vi "三个数中的最大最小数.vi"(1 "c":dbl, 2 "b":dbl, 3 "a":dbl) -> (0 "max":dbl)   [LabVIEW 2012]
doc: "功能：\n\n求给定三个数中的最大、最小值。\n\ncsxcs_366创建"
panel:
  out "min":dbl
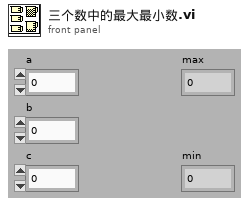
[diagram p1: front panel]
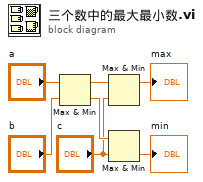
[diagram p0: block diagram]
diagram:
  n1 = Max & Min(x="a", y="b") -> (max(x,y)=w5:dbl, min(x,y)=w4:dbl)
  n2 = Max & Min(x=w5, y="c") -> (max(x,y)=→"max":dbl)  [unwired: 1 out]
  n3 = Max & Min(x=w4, y="c") -> (min(x,y)=→"min":dbl)  [unwired: 1 out]
